vi "finish.vi"(8 "ErrorIn":errorcluster, 11 "Queues":T1) -> (0 "ErrorOut":errorcluster)   [LabVIEW 2019]
uses:
  utilities/Queues.ctl
  GUIVIs/GUIInput.ctl
  MobileAnalyzer/mainVIs/UIVIs/AccelerationDataFrames.ctl
  GUIVIs/GUIOutput.ctl
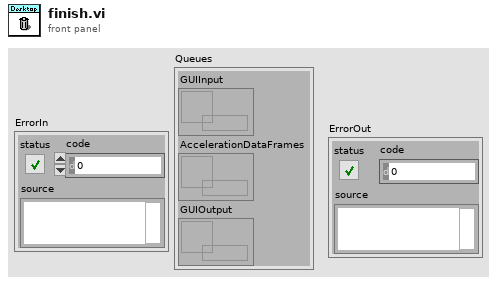
[diagram p1: front panel]
types:
  T1 = typedef "Queues.ctl" = cluster{"GUIInput":refnum<queue>, "AccelerationDataFrames":refnum<queue>, "GUIOutput":refnum<queue>}
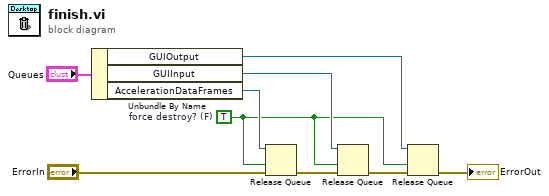
[diagram p0: block diagram]
diagram:
  w3 = TRUE  # force destroy? (F)
  n1 = Unbundle By Name("Queues") -> ("GUIOutput"=w2:refnum<queue>, "GUIInput"=w5:refnum<queue>, "AccelerationDataFrames"=w7:refnum<queue>)
  n2 = Release Queue(queue=w7, force destroy? (F)=w3, error in (no error)="ErrorIn") -> (error out=w6:errorcluster)  [unwired: 2 out]
  n3 = Release Queue(queue=w5, force destroy? (F)=w3, error in (no error)=w6) -> (error out=w4:errorcluster)  [unwired: 2 out]
  n4 = Release Queue(queue=w2, force destroy? (F)=w3, error in (no error)=w4) -> (error out=→"ErrorOut":errorcluster)  [unwired: 2 out]
